vi "Write_to_log.vi"(0 "TCP Refnum":refnum<k5>, 1 "Type":i8, 2 "Message":string, 3 "Cient ip":string) -> ()   [LabVIEW 2011]
doc: "The Ip adress and the date and time when the client logged in is stored to a log file located in *\\Serverlogs\\ServerEvents.log where * is the server dir . The date and time the server shuts down and starts is also stored by this vi."
uses:
  Server_Globals.vi
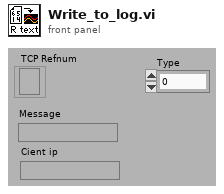
[diagram p1: front panel]
types:
  T1 = cluster{"Global":cluster{"Port":i32, "Reset Time":i32, "Maximum Delay":i32}, "Instrument Adress":cluster{"FGEN":string, "DC Power":string, "OSC":string, "USB":string, "DMM":string}, "Log":cluster{"Log Level":u32, "Log File":path}, "Digital Multimeter":cluster{"0":string, "1":string, "2":string, "3":string, "4":string}, "Function Generator":cluster{"0":string, "1":string, "2":string, "3":string, "4":string}, "Digital Osciliscope":cluster{"0":string, "1":string, "2":string, "3":string, "4":string}, "DC Power Supply":cluster{"0":string, "1":string, "2":string, "3":string, "4":string}, "USB Interface":cluster{"0":string, "1":string, "2":string, "3":string, "4":string}, "Components type":cluster{"Components type":string, "Components list":string}, "Matrix version":string, "Digital Multimeter Card 2":cluster{"0":string, "1":string, "2":string, "3":string, "4":string}}
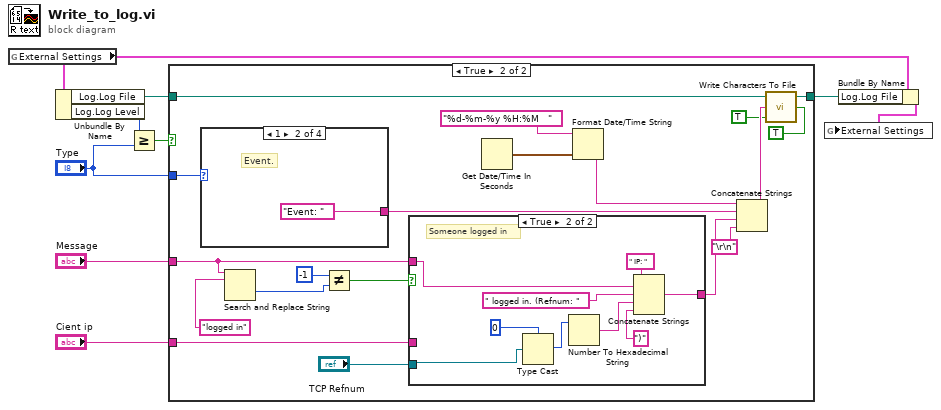
[diagram p0: block diagram]
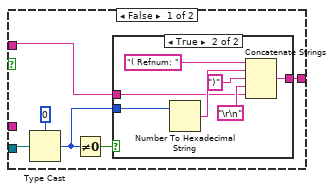
[diagram p3: hidden frame]
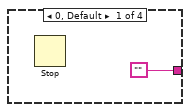
[diagram p5: hidden frame]
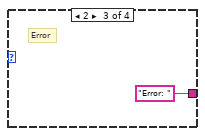
[diagram p6: hidden frame]
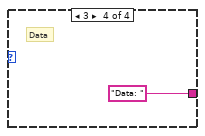
[diagram p7: hidden frame]
diagram:
  n1 = global read "Server_Globals.vi" "External Settings"() -> (w3:T1)
  n2 = Unbundle By Name(w3) -> ("Log.Log File"=w9:path, "Log.Log Level"=w8:u32)
  n3 = Greater Or Equal?(x=w8, y="Type") -> (x >= y?=w7:bool)
  n4 = case shown="True" w7 {
    tunnel: w9 -> [w10 w14]
    tunnel: "Message" -> [_ w24]
    tunnel: "Type" -> [_ w27]
    tunnel: "Cient ip" -> [_ w25]
    tunnel: [w10 w13] -> w2
    frame False {
    }
    frame True {
      n5 = case shown="1" w27 {
        tunnel: ["" "Event: " "Error: " "Data: "] -> w17
        frame 0, Default {
          n6 = Stop() -> ()  [unwired: 1 in]
        }
        frame 1 {
          # "Event."
        }
        frame 2 {
          # "Error"
        }
        frame 3 {
          # "Data"
        }
      }
      n7 = Search and Replace String(input string=w24, search string="logged in") -> (offset past replacement=w21:i32)  [unwired: 6 in, 3 out]
      n8 = Not Equal?(x=-1, y=w21) -> (x != y?=w20:bool)
      n9 = case shown="True" w20 {
        tunnel: [w32 w46] -> w16
        tunnel: "TCP Refnum" -> [w30 w44]
        tunnel: w25 -> [_ _]
        tunnel: w24 -> [w31 w45]
        frame False {
          n10 = Type Cast(type=0, x=w30) -> (*(type *) &x=w33:i32)
          n11 = Not Equal To 0?(x=w33) -> (x != 0?=w34:bool)
          n12 = case shown="True" w34 {
            tunnel: w31 -> [w36 w37]
            tunnel: [w36 w42] -> w32
            tunnel: w33 -> [_ w41]
            frame False {
            }
            frame True {
              n13 = Number To Hexadecimal String(2:w41) -> (0:w40:string)  [unwired: 1 in]
              n14 = Concatenate Strings("( Refnum: ", w40, ")", "\r\n", w37) -> (w42:string)
            }
          }
        }
        frame True {
          # "Someone logged in"
          n15 = Type Cast(type=0, x=w44) -> (*(type *) &x=w48:i32)
          n16 = Number To Hexadecimal String(2:w48) -> (0:w50:string)  [unwired: 1 in]
          n17 = Concatenate Strings(" IP: ", w45, " logged in. (Refnum: ", w50, ")") -> (w46:string)
        }
      }
      n18 = Get Date/Time In Seconds() -> (seconds since 1Jan1904=w28:timestamp)
      n19 = Format Date/Time String(time format string (%c)="%d-%m-%y %H:%M   ", seconds (now)=w28) -> (date/time string=w18:string)  [unwired: 1 in]
      n20 = Concatenate Strings(w18, w17, w16, "\r\n") -> (w15:string)
      n21 = call "Write Characters To File.vi"("convert eol? (no:F)"=TRUE ("convert eol (F)"), "append to file? (new file:F)"=TRUE, "character string"=w15, "file path (dialog if empty)"=w14) -> ("new file path (Not A Path if cancelled)"=w13:path)  [unwired: 1 out]
    }
  }
  n22 = Bundle By Name(cluster=w3, "Log.Log File"=w2) -> (w1:T1)
  n23 = global write "Server_Globals.vi" "External Settings"(w1) -> ()
